vi "LoadControlPanel.vi"(8 "error in (no error)":errorcluster, 10 "Actor In":refnum<class "Actor.lvclass">, 11 "DemoCamera in":refnum<class "DemoCamera.lvclass">) -> (0 "error out":errorcluster, 3 "DemoCamera out":refnum<class "DemoCamera.lvclass">)   [LabVIEW 2020, in "DemoCamera.lvlib" / "DemoCamera.lvclass"]
uses:
  DemoCamera.lvclass
  ViewController/Prime95BCameraController/CameraController.lvclass
  Hardware Abstraction Layer/Component/Camera/Camera/Camera.lvclass
  C:/Program Files/National Instruments/LabVIEW 2020/vi.lib/ActorFramework/Actor/Actor.lvclass
  <vilib>/ActorFramework/Actor/Actor.lvclass
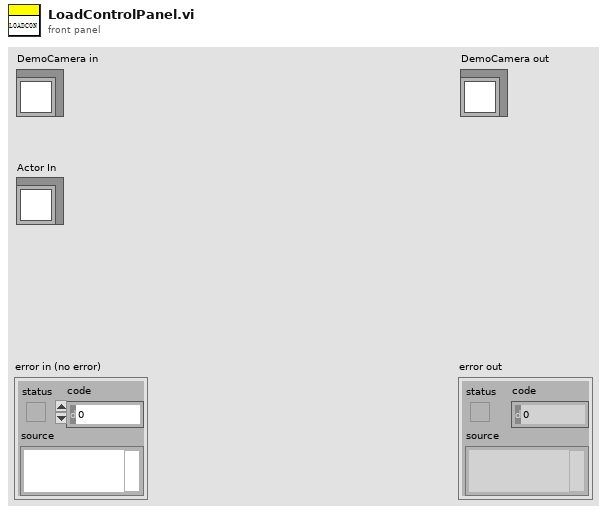
[diagram p1: front panel]
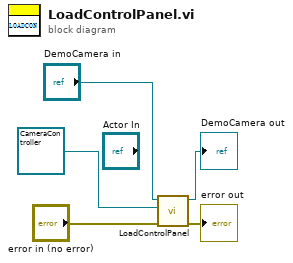
[diagram p0: block diagram]
diagram:
  n1 = call-parent "LoadControlPanel.vi"("error in (no error)"="error in (no error)", "Actor In"=refnum<class "CameraController.lvclass"> refnum ("Prime95BCameraController.lvlib:Prime95BCameraController.lvclass"), "GRMActor in"="DemoCamera in") -> ("error out"=→"error out":errorcluster, "GRMActor out"=→"DemoCamera out":refnum<class "DemoCamera.lvclass">)  [unwired: 7 in]
